vi "Filter_and_Chop (1 Ch).vi"(0 "Integrated Waveform":waveform(sgl)={"t0"=timestamp(0 s since 1904-01-01), "dt"=0.0, "Y"=[]}, 5 "Conversion Op":T1(ring), 9 "Channel Properties In":variant, 11 "error in (no error)":errorcluster) -> (3 "Filtered Waveform (unchopped)":waveform(sgl), 4 "Filtered and Chopped Waveform":waveform(sgl), 6 "Seconds Chopped Off":sgl, 8 "Data Valid?":bool=TRUE, 10 "Channel Properties Out":variant, 15 "error out":errorcluster)   [LabVIEW 2017, in "VibrationAnalysisFunctions.lvlib"]
uses:
  <vilib>/addons/InsightCM/Utilities/Analysis/Vibration/VibrationAnalysisFunctions.lvlib
  <vilib>/addons/Sound and Vibration/Order Analysis/Referece Data Processing/OAT IIR Preprocess Filter (1 Channel).vi
  <vilib>/addons/Sound and Vibration/Order Analysis/Referece Data Processing/SoundVib_RefDataProcess.lvlib
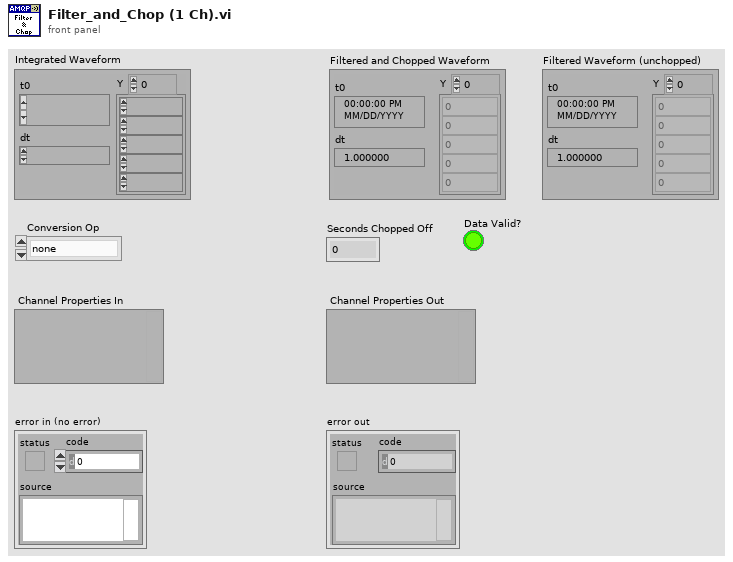
[diagram p1: front panel]
types:
  T1 = enum16{"none", "singleInt", "doubleInt", "singleDiff", "doubleDiff"}
  T2 = cluster{"low cutoff freq":dbl, "high cutoff freq":dbl}
  T3 = enum32{"Lowpass", "Highpass", "Bandpass", "Bandstop"}
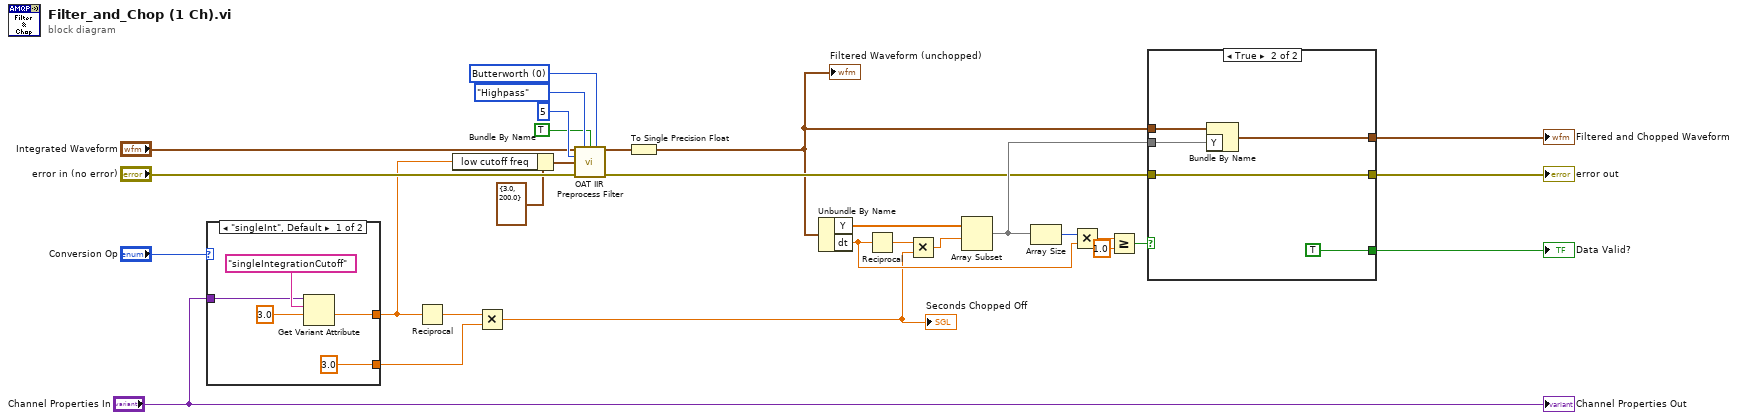
[diagram p0: block diagram]
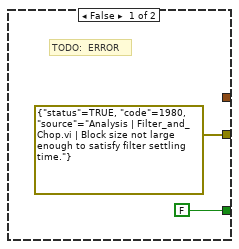
[diagram p2: hidden frame]
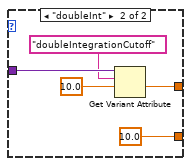
[diagram p3: hidden frame]
diagram:
  w28 = u16 0 items=["Butterworth", "Chebyshev", "Inverse Chebyshev", "Elliptic"] ("design method")
  n1 = case shown="\"singleInt\", Default" "Conversion Op" {
    tunnel: "Channel Properties In" -> [w33 w38]
    tunnel: [w32 w36] -> w18
    tunnel: [sgl 3.0 ("y") sgl 10.0 ("y")] -> w8
    frame "singleInt", Default {
      n2 = Get Variant Attribute(Variant=w33, name="singleIntegrationCutoff" ("Key"), default value (empty Variant)=sgl 3.0 ("low cutoff freq")) -> (value=w32:sgl)  [unwired: 1 in, 3 out]
    }
    frame "doubleInt" {
      n3 = Get Variant Attribute(Variant=w38, name="doubleIntegrationCutoff" ("Key"), default value (empty Variant)=sgl 10.0 ("low cutoff freq")) -> (value=w36:sgl)  [unwired: 1 in, 3 out]
    }
  }
  n4 = Reciprocal(x=w18) -> (1/x=w17:sgl)
  n5 = Bundle By Name(cluster=T2 {"low cutoff freq"=3.0, "high cutoff freq"=200.0} ("freq specs [Hz]"), "low cutoff freq"=w18) -> (w6:T2)
  n6 = Multiply(x=w17, y=w8) -> (x*y=w1:sgl)
  "Seconds Chopped Off" <- w1
  n7 = call-poly <vilib>:"OAT IIR Preprocess Filter.vi"("scaled signal [EU]"="Integrated Waveform", "filter type"=T3."Highpass", "reset? (F)"=TRUE, "design method"=w28, "order"=5, "freq specs [Hz]"=w6, "error in (no error)"="error in (no error)") -> ("filtered scaled signal [EU]"=w23:waveform(dbl), "error out"=w9:errorcluster)  [unwired: 7 in]
  n8 = To Single Precision Float(number=w23) -> (single precision float=w4:waveform(sgl))
  "Filtered Waveform (unchopped)" <- w4
  n9 = Unbundle By Name(w4) -> ("Y"=w25:sgl[], "dt"=w14:dbl)
  n10 = Reciprocal(x=w14) -> (1/x=w22:dbl)
  n11 = Multiply(x=w22, y=w1) -> (x*y=w16:dbl)
  n12 = Array Subset(array=w25, index=w16) -> (w10:sgl[])  [unwired: 1 in]
  n13 = Array Size(array=w10) -> (size(s)=w15:i32)
  n14 = Multiply(x=w15, y=w14) -> (x*y=w13:dbl)
  n15 = Greater Or Equal?(x=w13, y=1.0) -> (x >= y?=w11:bool)
  n16 = case shown="True" w11 {
    tunnel: w4 -> [_ w46]
    tunnel: w10 -> [_ w45]
    tunnel: [_ w44] -> w3
    tunnel: w9 -> [_ w43]
    tunnel: [errorcluster {"status"=TRUE, "code"=1980, "source"="Analysis | Filter_and_Chop.vi | Block size not large enough to satisfy filter settling time."} ("error out") w43] -> w2
    tunnel: [FALSE ("reset? (F)") TRUE ("reset? (F)")] -> w7
    frame False {
      # "TODO:  ERROR"
    }
    frame True {
      n17 = Bundle By Name(cluster=w46, "Y"=w45) -> (w44:waveform(sgl))
    }
  }
  "Filtered and Chopped Waveform" <- w3
  "error out" <- w2
  "Data Valid?" <- w7
  "Channel Properties Out" <- "Channel Properties In"
